vi "SEARCH_lines_io.vi"(8 "IN str":string, 11 "Array define":string[][](array[string])) -> (3 "OUT lines":string)   [LabVIEW 2017]
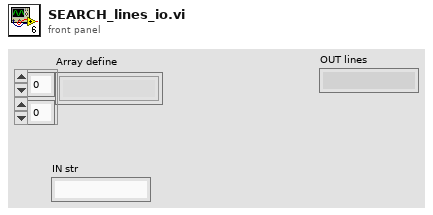
[diagram p1: front panel]
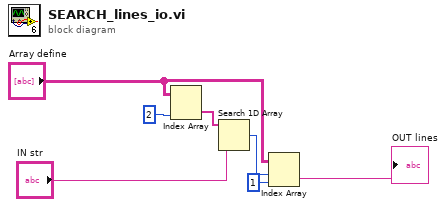
[diagram p0: block diagram]
diagram:
  n1 = Index Array(array="Array define", index (col)=2 ("disabled index (col)")) -> (element=w5:string[])  [unwired: 1 in]
  n2 = Search 1D Array(1D array=w5, element="IN str") -> (index of element=w6:i32)  [unwired: 1 in]
  n3 = Index Array(array="Array define", index (row)=w6, index (col)=1 ("disabled index (col)")) -> (element=→"OUT lines":string)
